vi "Z_ROI_compiler-Adjust for short acquisition cycles.vi"(0 "Number of POIs":i32, 1 "Cycle time (us)":dbl, 2 "dISABLE":bool, 5 "Total number of miniscans":i32, 7 "Number of cycles":u64, 9 "ROI Attributes":T1[](array[typedef]) {"ROI group ID" format="%#_6f"; "Laser Power (%)" format="%#_6f"; "Zoom" format="%#_6f"; "Frame Size" format="%#_6f"; "Number of lines" format="%#_6f"; "Composite ID" format="%#_6f"; "Angle (deg)" format="%#_6f"; "ROI Time (ns)" format="%#_6f"; "ROI ID" format="%#_6f"; "Pixels in ROI" format="%#_6f"; "ROI index" format="%#_6f"; "Z stop" format="%#_6f"; "Y stop" format="%#_6f"; "X stop" format="%#_6f"; "Z start" format="%#_6f"; "X start" format="%#_6f"; "Y start" format="%#_6f"}, 11 "ROI Attributes (broken down to miniscans) in":T1[](array[typedef]) {"ROI group ID" format="%#_6f"; "Laser Power (%)" format="%#_6f"; "Zoom" format="%#_6f"; "Frame Size" format="%#_6f"; "Number of lines" format="%#_6f"; "Composite ID" format="%#_6f"; "Angle (deg)" format="%#_6f"; "ROI Time (ns)" format="%#_6f"; "ROI ID" format="%#_6f"; "Pixels in ROI" format="%#_6f"; "ROI index" format="%#_6f"; "Z stop" format="%#_6f"; "Y stop" format="%#_6f"; "X stop" format="%#_6f"; "Z start" format="%#_6f"; "X start" format="%#_6f"; "Y start" format="%#_6f"}, 12 "ROI Coordinates (broken down to miniscans) in":T2, 13 "Zoom":dbl[](array[numeric])) -> (3 "Cycle time (us) (multiplied by number of stacked cycles)":dbl, 4 "Number of POIs (multiplied by number of stacked cycles)":i32, 6 "Number of miniscans (multiplied by number of stacked cycles)":i32, 8 "Number of cycles or number of stacked cycles":u64, 10 "Zoom":dbl[](array[numeric]), 14 "ROI Coordinates (broken down to miniscans) out":T2, 15 "ROI Attributes (broken down to miniscans) out":T1[](array[typedef]) {"ROI group ID" format="%#_6f"; "Laser Power (%)" format="%#_6f"; "Zoom" format="%#_6f"; "Frame Size" format="%#_6f"; "Number of lines" format="%#_6f"; "Composite ID" format="%#_6f"; "Angle (deg)" format="%#_6f"; "ROI Time (ns)" format="%#_6f"; "ROI ID" format="%#_6f"; "Pixels in ROI" format="%#_6f"; "ROI index" format="%#_6f"; "Z stop" format="%#_6f"; "Y stop" format="%#_6f"; "X stop" format="%#_6f"; "Z start" format="%#_6f"; "X start" format="%#_6f"; "Y start" format="%#_6f"})   [LabVIEW 2017]
uses:
  User Interface/Visualisation/Functional Imaging Viewer/Typedefs/ROI parameters data type.ctl
  Typedefs/ROI XY coordinates cluster.ctl
panel:
  in  "Acquisition length (sec)":dbl
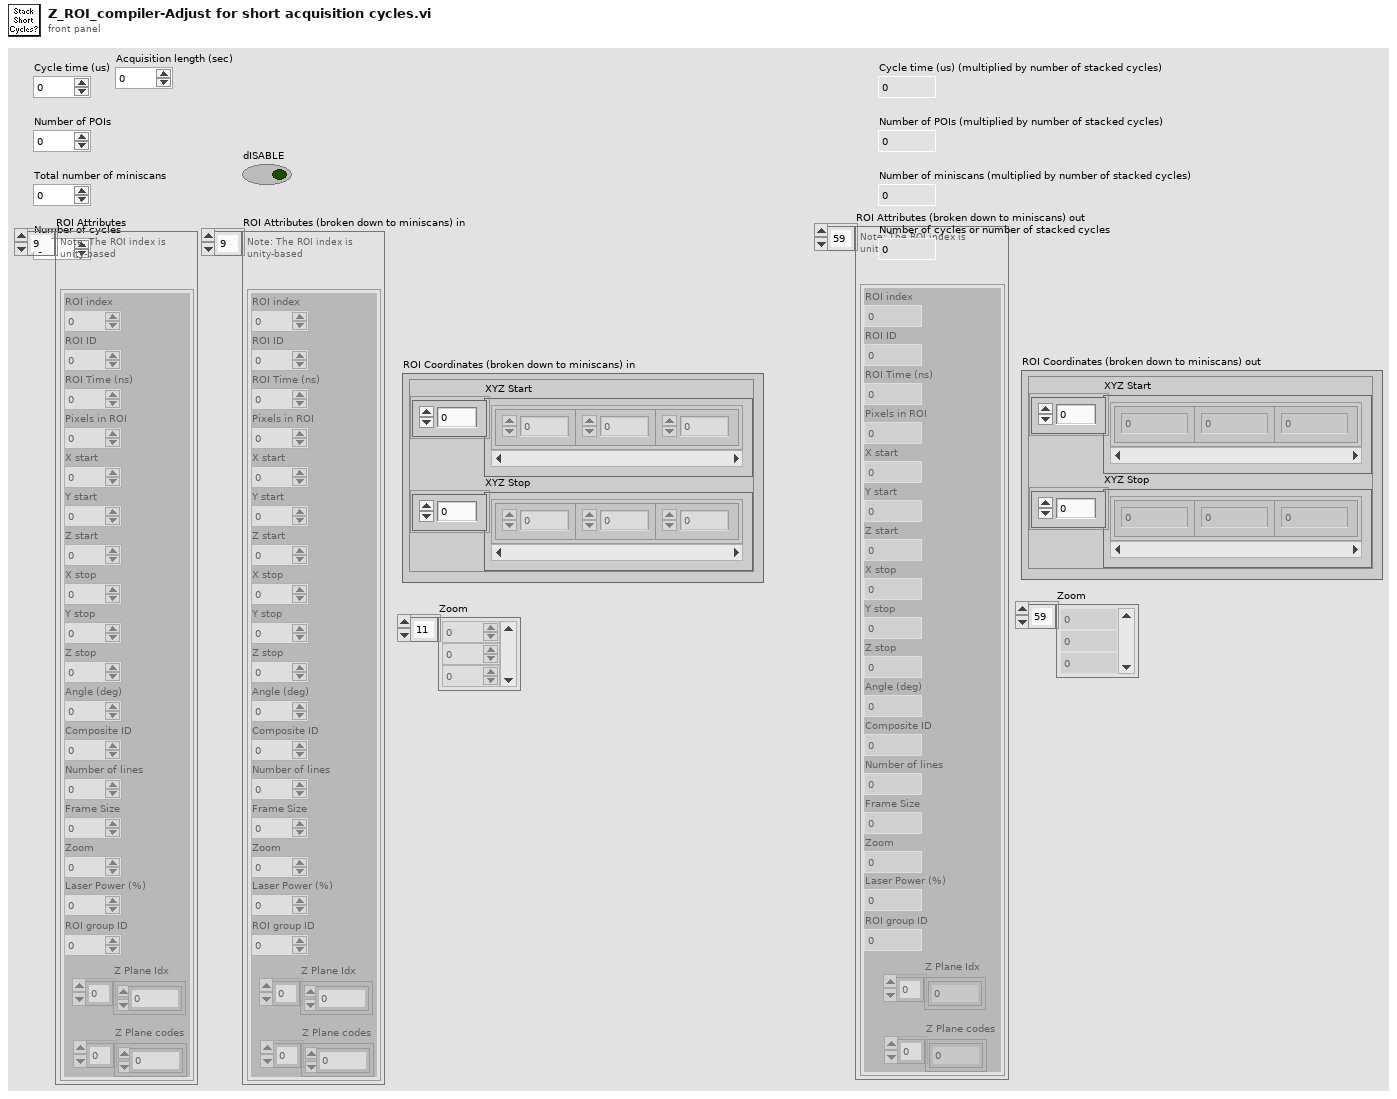
[diagram p1: front panel]
types:
  T1 = typedef "ROI parameters data type.ctl" = cluster{"ROI index":dbl, "ROI ID":dbl, "ROI Time (ns)":dbl, "Pixels in ROI":dbl, "X start":dbl, "Y start":dbl, "Z start":dbl, "X stop":dbl, "Y stop":dbl, "Z stop":dbl, "Angle (deg)":dbl, "Composite ID":dbl, "Number of lines":dbl, "Frame Size":dbl, "Zoom":dbl, "Laser Power (%)":dbl, "ROI group ID":dbl, "Z Plane Idx":i32[], "Z Plane codes":i32[]}
  T2 = typedef "ROI XY coordinates cluster.ctl" = cluster{"XYZ Start":cluster{"X":sgl, "Y":sgl, "Z":sgl}[], "XYZ Stop":cluster{"X":sgl, "Y":sgl, "Z":sgl}[]}
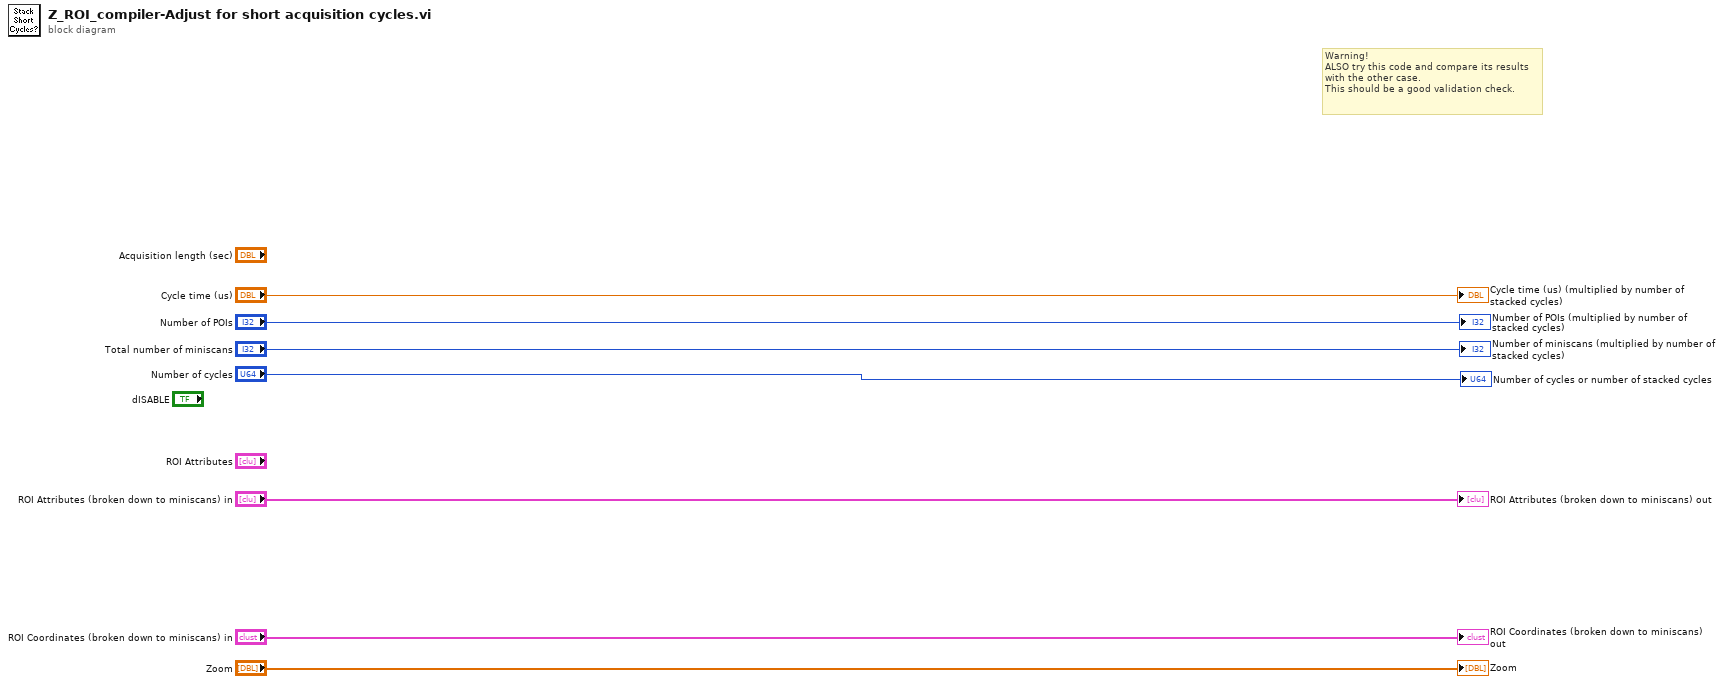
[diagram p0: block diagram]
diagram:
  # "Warning!\nALSO try this code and compare its results with the other case.\nThis should be a good validation check."
  "ROI Attributes (broken down to miniscans) out" <- "ROI Attributes (broken down to miniscans) in"
  "ROI Coordinates (broken down to miniscans) out" <- "ROI Coordinates (broken down to miniscans) in"
  "Cycle time (us) (multiplied by number of stacked cycles)" <- "Cycle time (us)"
  "Number of miniscans (multiplied by number of stacked cycles)" <- "Total number of miniscans"
  "Number of POIs (multiplied by number of stacked cycles)" <- "Number of POIs"
  "Number of cycles or number of stacked cycles" <- "Number of cycles"
  "Zoom" <- "Zoom"
